vi "Step Trigger VI.vi"(8 "error in (no error)":errorcluster, 11 "SDF path":path) -> (0 "error out":errorcluster)   [LabVIEW 2019, in "TimingDRV System Explorer.lvlib"]
uses:
  TimingDRV System Explorer.lvlib
panel:
  out "Target IP Address":string
  out "Connected?":bool
  in  "Switch Automated":bool
  in  "Switch Manual":bool
  in  "Exit":bool
  in  "Send Trigger":bool
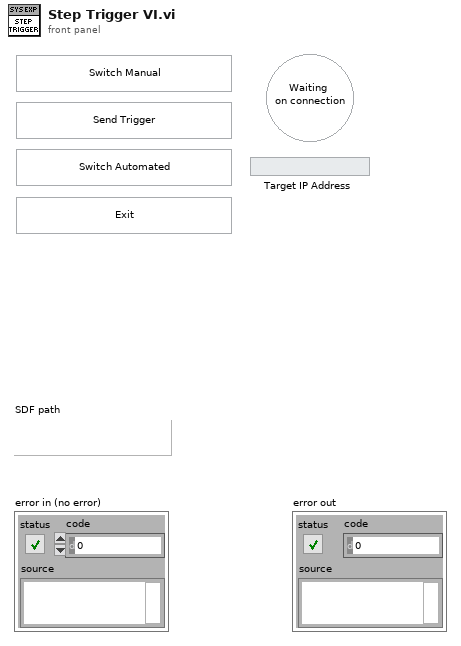
[diagram p1: front panel]
types:
  T1 = enum32{"Invalid", "Standard", "Closed", "Hidden", "Minimized", "Maximized"}
  T2 = enum16{"Always On", "Always Off", "Off While Running"}
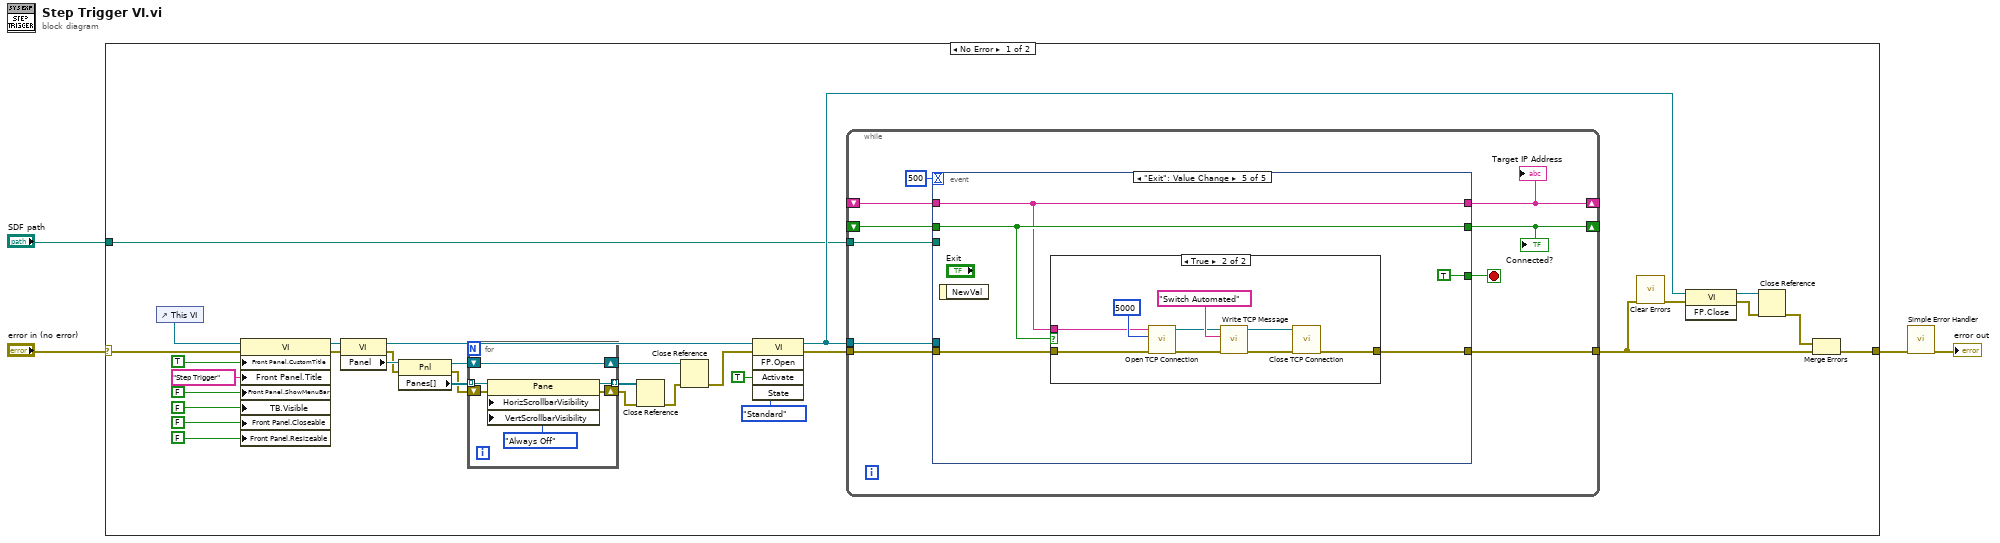
[diagram p0: block diagram]
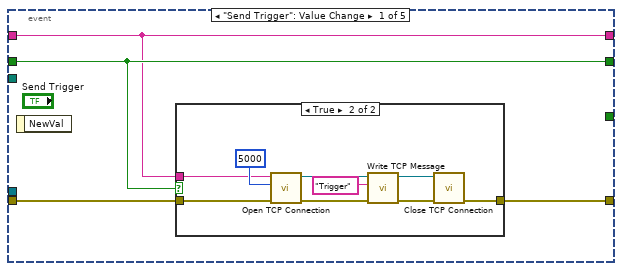
[diagram p2: hidden frame]
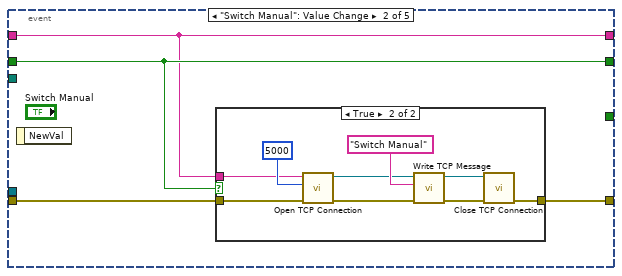
[diagram p4: hidden frame]
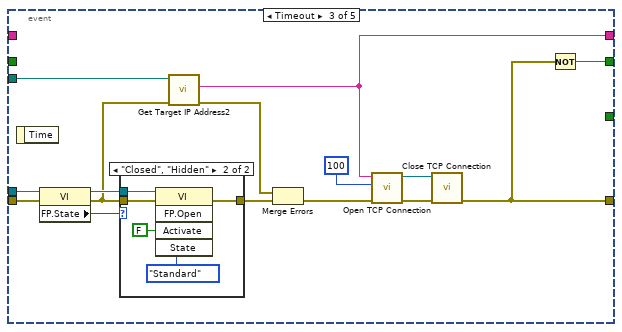
[diagram p6: hidden frame]
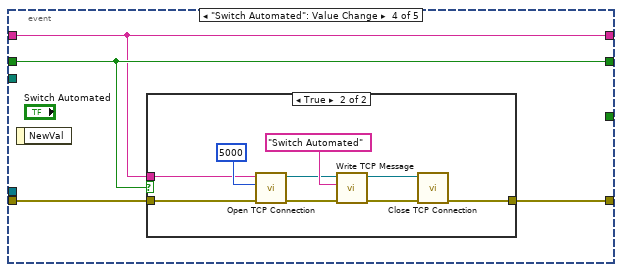
[diagram p8: hidden frame]
diagram:
  n1 = case shown="No Error" "error in (no error)" {
    selector: "error in (no error)" -> [w30 w131]
    tunnel: [w36 w131] -> w3
    tunnel: "SDF path" -> [w6 _]
    frame No Error {
      n2 = control-ref of="This VI"() -> (w29:refnum<vi>)
      n3 = property class="VI"(reference=w29, error in=w30, "Front Panel.CustomTitle"=TRUE ("Front Panel Window:Custom Title"), "Front Panel.Title"="Step Trigger" ("Front Panel Window:Title"), "Front Panel.ShowMenuBar"=FALSE ("Front Panel Window:Show Menu Bar"), "TB.Visible"=FALSE ("Tool Bar:Visible"), "Front Panel.Closeable"=FALSE ("Front Panel Window:Closeable"), "Front Panel.Resizeable"=FALSE ("Front Panel Window:Resizable")) -> (reference out=w19:refnum<vi>, error out=w18:errorcluster)
      n4 = property class="VI"(reference=w19, error in=w18) -> (reference out=w8:refnum<vi>, error out=w12:errorcluster, "Panel"=w17:refnum<vi>)
      n5 = property class="Pnl"(reference=w17, error in=w12) -> (reference out=w14:refnum<vi>, error out=w11:errorcluster, "Panes[]"=w16:refnum<vi>[])
      n6 = for {
        tunnel: w16 -> [w42] mode=indexing
        tunnel: [w40] -> w15 mode=indexing
        shift-right: [w39] -> w13
        shift-left: w14 -> [w39]
        shift-right: [w37] -> w10
        shift-left: w11 -> [w38]
        w41 = T2."Always Off" ("Horizontal Scrollbar Visibility")
        n7 = property class="Pane"(reference=w42, error in=w38, "HorizScrollbarVisibility"=w41, "VertScrollbarVisibility"=w41) -> (reference out=w40:refnum<vi>, error out=w37:errorcluster)
      }
      n8 = Close Reference(reference=w15, error in (no error)=w10) -> (error out=w9:errorcluster)
      n9 = Close Reference(reference=w13, error in (no error)=w9) -> (error out=w7:errorcluster)
      n10 = invoke class="VI" method="FP.Open"(reference=w8, error in=w7, "Activate"=TRUE ("Activate?"), "State"=T1."Standard") -> (reference out=w23:refnum<vi>, error out=w32:errorcluster)  [unwired: 1 in, 3 out]
      n11 = while {
        tunnel: [w50] -> w31
        tunnel: w32 -> [w49]
        tunnel: w23 -> [w48]
        tunnel: w6 -> [w47]
        shift-right: [w45] -> _
        shift-left: _ -> [w46]
        shift-right: [w43] -> _
        shift-left: _ -> [w44]
        stop <- w52 stop-if-true
        n12 = event shown="[4] \"Exit\": Value Change" {
          selector: _ -> [_ _ _ _ _]
          dyn-events: _ -> [_ _ _ _ _]
          timeout: 500 -> [_ _ _ _ _]
          tunnel: [_ _ _ _ TRUE ("Stop")] -> w52
          tunnel: [w56 w70 w95 w105 w118] -> w50
          tunnel: w49 -> [w55 w69 w86 w104 w119]
          tunnel: w48 -> [_ _ w87 _ _]
          tunnel: w47 -> [_ _ w91 _ _]
          tunnel: w46 -> [w53 w67 _ w102 w116]
          tunnel: [w53 w67 w82 w102 w116] -> w45
          tunnel: [w54 w68 w81 w103 w117] -> w43
          tunnel: w44 -> [w54 w68 _ w103 w117]
          event "Send Trigger": Value Change {
            n13 = event-data() -> ()  [unwired: 1 in, 1 out]
            n14 = case shown="True" w54 {
              tunnel: [w57 w60] -> w56
              tunnel: w55 -> [w57 w59]
              tunnel: w53 -> [_ w58]
              frame False {
              }
              frame True {
                n15 = call "Open TCP Connection.vi"("error in (no error)"=w59, "timeout ms (60000)"=5000, "network address"=w58) -> ("error out"=w65:errorcluster, "TCP Network Connection out"=w64:refnum<k5>)  [unwired: 7 in]
                n16 = call "Write TCP Message.vi"("error in (no error)"=w65, "Message (string)"="Trigger" ("Trigger"), "TCP Network Connection in"=w64) -> ("error out"=w63:errorcluster, "TCP Network Connection out"=w62:refnum<k5>)  [unwired: 7 in]
                n17 = call "Close TCP Connection.vi"("error in (no error)"=w63, "TCP Network Connection in"=w62) -> ("error out"=w60:errorcluster)  [unwired: 9 in]
              }
            }
          }
          event "Switch Manual": Value Change {
            n18 = event-data() -> ()  [unwired: 1 in, 1 out]
            n19 = case shown="True" w68 {
              tunnel: [w71 w74] -> w70
              tunnel: w69 -> [w71 w73]
              tunnel: w67 -> [_ w72]
              frame False {
              }
              frame True {
                n20 = call "Open TCP Connection.vi"("error in (no error)"=w73, "timeout ms (60000)"=5000, "network address"=w72) -> ("error out"=w77:errorcluster, "TCP Network Connection out"=w75:refnum<k5>)  [unwired: 7 in]
                n21 = call "Write TCP Message.vi"("error in (no error)"=w77, "Message (string)"="Switch Manual" ("Switch Manual"), "TCP Network Connection in"=w75) -> ("error out"=w79:errorcluster, "TCP Network Connection out"=w78:refnum<k5>)  [unwired: 7 in]
                n22 = call "Close TCP Connection.vi"("error in (no error)"=w79, "TCP Network Connection in"=w78) -> ("error out"=w74:errorcluster)  [unwired: 9 in]
              }
            }
          }
          event Timeout {
            n23 = event-data() -> ()  [unwired: 1 in, 1 out]
            n24 = property class="VI"(reference=w87, error in=w86) -> (reference out=w84:refnum<vi>, error out=w83:errorcluster, "FP.State"=w85:T1)
            n25 = case shown="\"Closed\", \"Hidden\"" w85 {
              tunnel: [w96 w100] -> w90
              tunnel: w83 -> [w96 w98]
              tunnel: w84 -> [_ w97]
              frame "Invalid", Default {
              }
              frame "Closed", "Hidden" {
                n26 = invoke class="VI" method="FP.Open"(reference=w97, error in=w98, "Activate"=FALSE ("Activate?"), "State"=T1."Standard") -> (error out=w100:errorcluster)  [unwired: 1 in, 4 out]
              }
            }
            n27 = call "Get Target IP Address2.vi"("error in (no error)"=w83, "SDF path"=w91) -> ("error out"=w89:errorcluster, "target ip address"=w82:string)  [unwired: 8 in]
            n28 = Merge Errors(w89, w90) -> (w88:errorcluster)
            n29 = call "Open TCP Connection.vi"("error in (no error)"=w88, "timeout ms (60000)"=100, "network address"=w82) -> ("error out"=w94:errorcluster, "TCP Network Connection out"=w93:refnum<k5>)  [unwired: 7 in]
            n30 = call "Close TCP Connection.vi"("error in (no error)"=w94, "TCP Network Connection in"=w93) -> ("error out"=w95:errorcluster)  [unwired: 9 in]
            n31 = Not(x=w95) -> (.not. x?=w81:bool)
          }
          event "Switch Automated": Value Change {
            n32 = event-data() -> ()  [unwired: 1 in, 1 out]
            n33 = case shown="True" w103 {
              tunnel: [w106 w109] -> w105
              tunnel: w104 -> [w106 w108]
              tunnel: w102 -> [_ w107]
              frame False {
              }
              frame True {
                n34 = call "Open TCP Connection.vi"("error in (no error)"=w108, "timeout ms (60000)"=5000, "network address"=w107) -> ("error out"=w114:errorcluster, "TCP Network Connection out"=w112:refnum<k5>)  [unwired: 7 in]
                n35 = call "Write TCP Message.vi"("error in (no error)"=w114, "Message (string)"="Switch Automated" ("Switch Automated"), "TCP Network Connection in"=w112) -> ("error out"=w111:errorcluster, "TCP Network Connection out"=w110:refnum<k5>)  [unwired: 7 in]
                n36 = call "Close TCP Connection.vi"("error in (no error)"=w111, "TCP Network Connection in"=w110) -> ("error out"=w109:errorcluster)  [unwired: 9 in]
              }
            }
          }
          event "Exit": Value Change {
            n37 = event-data() -> ()  [unwired: 1 in, 1 out]
            n38 = case shown="True" w117 {
              tunnel: [w121 w124] -> w118
              tunnel: w119 -> [w121 w123]
              tunnel: w116 -> [_ w122]
              frame False {
              }
              frame True {
                n39 = call "Open TCP Connection.vi"("error in (no error)"=w123, "timeout ms (60000)"=5000, "network address"=w122) -> ("error out"=w129:errorcluster, "TCP Network Connection out"=w127:refnum<k5>)  [unwired: 7 in]
                n40 = call "Write TCP Message.vi"("error in (no error)"=w129, "Message (string)"="Switch Automated" ("Switch Automated"), "TCP Network Connection in"=w127) -> ("error out"=w126:errorcluster, "TCP Network Connection out"=w125:refnum<k5>)  [unwired: 7 in]
                n41 = call "Close TCP Connection.vi"("error in (no error)"=w126, "TCP Network Connection in"=w125) -> ("error out"=w124:errorcluster)  [unwired: 9 in]
              }
            }
          }
        }
        "Target IP Address" <- w45
        "Connected?" <- w43
      }
      n42 = call <vilib>:"Clear Errors.vi"("error in (no error)"=w31) -> ("error out"=w35:errorcluster)  [unwired: 5 in, 1 out]
      n43 = invoke class="VI" method="FP.Close"(reference=w23, error in=w35) -> (reference out=w20:refnum<vi>, error out=w22:errorcluster)  [unwired: 1 in, 1 out]
      n44 = Close Reference(reference=w20, error in (no error)=w22) -> (error out=w21:errorcluster)
      n45 = Merge Errors(w21, w31) -> (w36:errorcluster)
    }
    frame Error {
    }
  }
  n46 = call <vilib>:"Simple Error Handler.vi"("error in (no error)"=w3) -> ("error out"=→"error out":errorcluster)  [unwired: 4 in, 4 out]
